vi "Identities.vi"(8 "error in (no error)":errorcluster, 11 "AbortManagerAPI in":refnum<class "AbortManagerAPI.lvclass">) -> (0 "error out":errorcluster, 2 "Identities":refnum<class "Identity.lvclass">[](array[class]), 3 "AbortManagerAPI out":refnum<class "AbortManagerAPI.lvclass">)   [LabVIEW 2020, in "Volatus.lvlib" / "AbortManagerAPI.lvclass"]
uses:
  AbortManagerAPI.lvclass
  Identity/Identity.lvclass
  AbortManagerAPI.lvclass/AbortManagerAPI.ctl
  AbortManagerIdentity/AbortManagerIdentity.lvclass
  C:/dev/lv20CE/relink/lv-volatus/Volatus/AbortManagerIdentity/AbortManagerIdentity.lvclass
  C:/dev/lv20CE/relink/lv-volatus/Volatus/Identity/Identity.lvclass
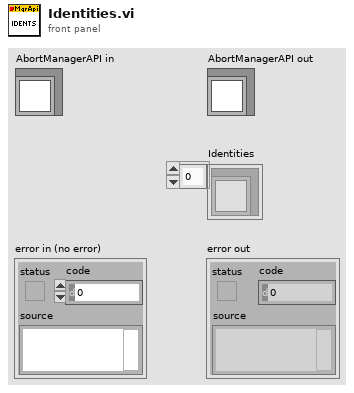
[diagram p1: front panel]
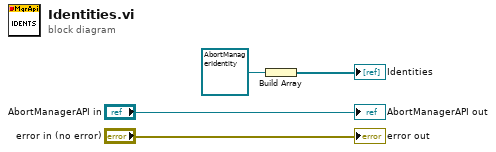
[diagram p0: block diagram]
diagram:
  n1 = Build Array(refnum<class "AbortManagerIdentity.lvclass"> refnum ("Volatus:AbortManagerIdentity.lvclass")) -> (→"Identities":refnum<class "AbortManagerIdentity.lvclass">[])
  "error out" <- "error in (no error)"
  "AbortManagerAPI out" <- "AbortManagerAPI in"
